vi "does_plane_hit.vi"(8 "error in (no error)":errorcluster, 9 "depth":dbl[unit], 11 "Box in":refnum<class "Box.lvclass">) -> (0 "error out":errorcluster, 2 "is inside?":bool, 3 "Box out":refnum<class "Box.lvclass">)   [LabVIEW 2010, in "Box.lvclass"]
uses:
  Box.lvclass
  SpaceVector/SpaceVector/SpaceVector.lvclass
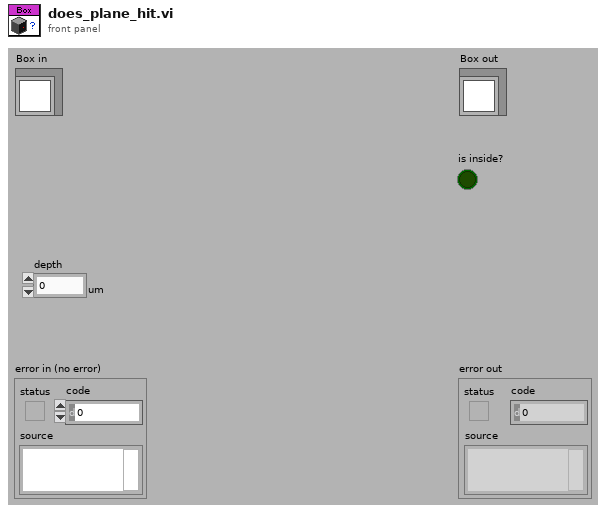
[diagram p1: front panel]
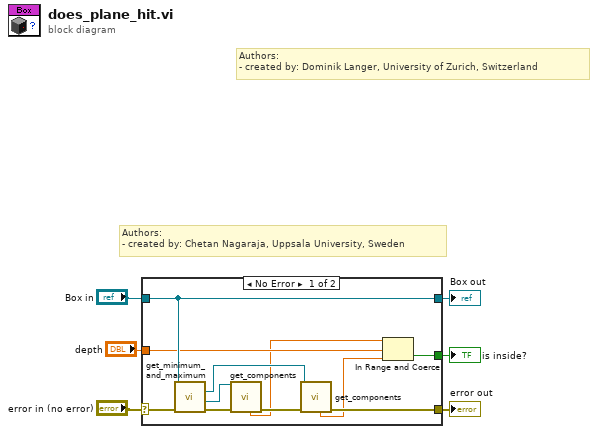
[diagram p0: block diagram]
diagram:
  # "Authors: \n- created by: Chetan Nagaraja, Uppsala University, Sweden"
  # "Authors: \n- created by: Dominik Langer, University of Zurich, Switzerland"
  n1 = case shown="No Error" "error in (no error)" {
    selector: "error in (no error)" -> [w16 w19]
    tunnel: [w11 w19] -> w5
    tunnel: [w17 w18] -> w3
    tunnel: "Box in" -> [w17 w18]
    tunnel: "depth" -> [w13 _]
    tunnel: [w7 _] -> w1
    frame No Error {
      n2 = call "get_minimum_and_maximum.vi"("error in (no error)"=w16, "Box in"=w17) -> ("error out"=w15:errorcluster, "maximum"=w14:refnum<class "SpaceVector.lvclass">, "minimum"=w10:refnum<class "SpaceVector.lvclass">)  [unwired: 6 in, 1 out]
      n3 = call "get_components.vi"("error in (no error)"=w15, "SpaceVector in"=w14) -> ("error out"=w12:errorcluster, "z"=w9:dbl[unit])  [unwired: 4 in, 4 out]
      n4 = call "get_components.vi"("error in (no error)"=w12, "SpaceVector in"=w10) -> ("error out"=w11:errorcluster, "z"=w8:dbl[unit])  [unwired: 4 in, 4 out]
      n5 = In Range and Coerce(upper limit=w9, x=w13, lower limit=w8) -> (In Range?=w7:bool)  [unwired: 1 out]
    }
    frame Error {
    }
  }
  "error out" <- w5
  "Box out" <- w3
  "is inside?" <- w1
